vi "read station lvdt precision config.vi"(8 "error in":errorcluster, 10 "station":string, 11 "configuration file path in":path) -> (0 "error out":errorcluster, 2 "lvdt precision":T1, 3 "configuration file path out":path)   [LabVIEW 2018]
uses:
  05.UserVI's/LVDT's/lvdt precision.ctl
  05.UserVI's/file io/ini/type defs/ini file actions.ctl
  05.UserVI's/file io/ini/type defs/ini entry value.ctl
  05.UserVI's/file io/ini/type defs/ini entry types.ctl
  05.UserVI's/file io/ini/type defs/ini entry.ctl
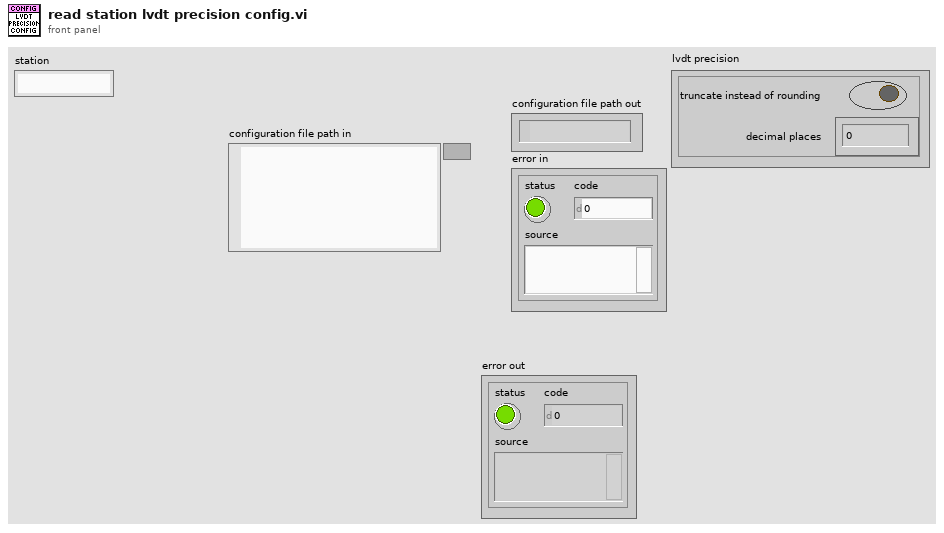
[diagram p1: front panel]
types:
  T1 = typedef "lvdt precision.ctl" = cluster{"truncate instead of rounding":bool, "decimal places":u8}
  T2 = typedef "ini entry value.ctl" = cluster{"Boolean":bool, "Dbl":dbl, "I32":i32, "Path":path, "String":string, "U32":u32}
  T3 = typedef "ini file actions.ctl" = enum16{"read ini", "write ini"}
  T4 = typedef "ini entry.ctl" = cluster{"section":string, "key":string, "type":T5, "default value":T2}
  T5 = typedef "ini entry types.ctl" = enum16{"Boolean", "Double", "I32", "Path", "String", "U32"}
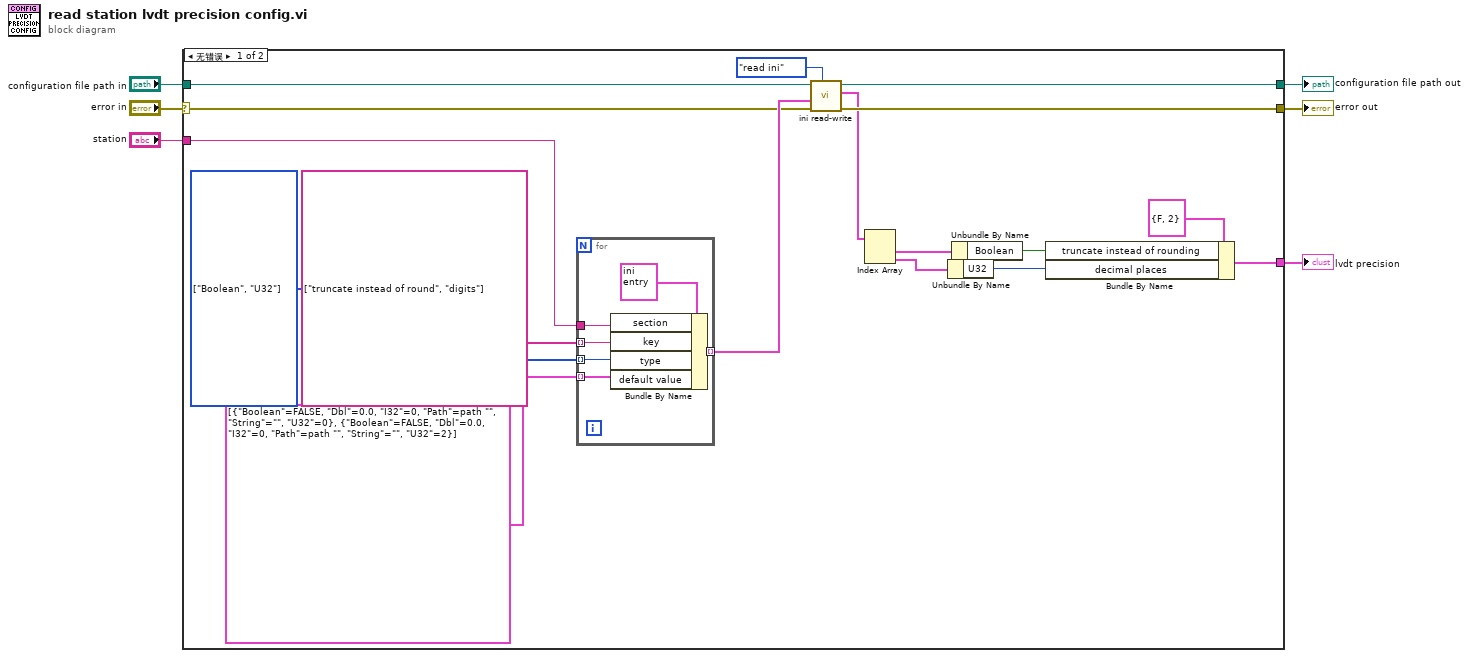
[diagram p0: block diagram]
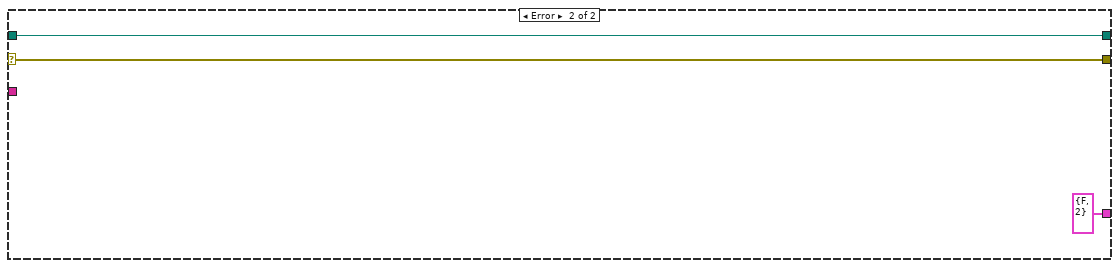
[diagram p2: hidden frame]
diagram:
  n1 = case shown="无错误" "error in" {
    selector: "error in" -> [w16 w32]
    tunnel: "configuration file path in" -> [w23 w31]
    tunnel: [w21 w31] -> w5
    tunnel: [w15 w32] -> w4
    tunnel: "station" -> [w14 _]
    tunnel: [w7 T1 {"truncate instead of rounding"=FALSE, "decimal places"=2} ("lvdt precision")] -> w1
    frame No Error {
      w19 = T5[] [enum."Boolean", enum."U32"] items=["Boolean", "Double", "I32", "Path", "String", "U32"]
      n2 = for {
        tunnel: w14 -> [w28]
        tunnel: string[] ["truncate instead of round", "digits"] -> [w27] mode=indexing
        tunnel: w19 -> [w26] mode=indexing
        tunnel: T2[] [{"Boolean"=FALSE, "Dbl"=0.0, "I32"=0, "Path"=path "", "String"="", "U32"=0}, {"Boolean"=FALSE, "Dbl"=0.0, "I32"=0, "Path"=path "", "String"="", "U32"=2}] -> [w25] mode=indexing
        tunnel: [w24] -> w17 mode=indexing
        n3 = Bundle By Name(cluster=T4 {"section"="", "key"="", "type"=enum."Boolean", "default value"={"Boolean"=FALSE, "Dbl"=0.0, "I32"=0, "Path"=path "", "String"="", "U32"=0}}, "section"=w28, "key"=w27, "type"=w26, "default value"=w25) -> (w24:T4)
      }
      n4 = call "ini read-write.vi"("action"=ini_file_actions."read ini", "error in (no error)"=w16, "ini entry descriptors"=w17, "configuration file path"=w23) -> ("error out"=w15:errorcluster, "values out"=w13:T2[], "configuration file path out"=w21:path)  [unwired: 5 in]
      n5 = Index Array(array=w13) -> (element #1=w12:T2, element #2=w11:T2)  [unwired: 2 in]
      n6 = Unbundle By Name(w11) -> ("U32"=w9:u32)
      n7 = Unbundle By Name(w12) -> ("Boolean"=w8:bool)
      n8 = Bundle By Name(cluster=T1 {"truncate instead of rounding"=FALSE, "decimal places"=2} ("lvdt precision"), "truncate instead of rounding"=w8, "decimal places"=w9) -> (w7:T1)
    }
    frame Error {
    }
  }
  "configuration file path out" <- w5
  "error out" <- w4
  "lvdt precision" <- w1
